vi "Trigger AI Acquisition.vi"() -> ()   [LabVIEW 2015]
doc: "이 예는 DAQmx 디바이스를 사용하여 버퍼링된 전압 측정을 연속적으로 수집하는 방법을 보여줍니다.\n\nDAQ 디바이스에 신호를 연결하는 방법에 대한 설명은 해당 디바이스 문서를 참조하십시오."
uses:
  <vilib>/DAQmx/read.llb/DAQmx Read (Analog 1D Wfm NChan NSamp).vi
  <vilib>/DAQmx/create/channels.llb/DAQmx Create Channel (AI-Voltage-Basic).vi
  <vilib>/DAQmx/configure/timing.llb/DAQmx Timing (Sample Clock).vi
  <vilib>/DAQmx/configure/task.llb/DAQmx Configure Logging (TDMS).vi
  <vilib>/DAQmx/configure/trigger.llb/DAQmx Start Trigger (Digital Edge).vi
  <vilib>/DAQmx/miscellaneous.llb/DAQmx Fill In Error Info.vi
  <resource>/objmgr/daqmx.rc
panel:
  in  "에지":i32(ring)=10280 items=["상승"=10280, "하강"=10171]
  in  "소스":tag
  in  "정지":bool
  out "웨이브폼 그래프":waveform(dbl)[](graph)
  in  "TDMS파일 경로":path
  in  "루프당 샘플":i32=1000
  in  "샘플 속도":dbl=1000.0
  in  "샘플 클럭 소스":tag="OnboardClock"
  in  "터미널 설정":i32(ring)=-1 items=["기본"=-1, "RSE"=10083, "NRSE"=10078, "차동"=10106, "유사 차동"=12529]
  in  "최대 전압":dbl=5.0
  in  "최소 전압":dbl=-5.0
  in  "물리적 채널":tag="Dev1/ai0"
  out "실제 샘플 속도":dbl=1000.0 format="%0.2f"
  in  "로깅 모드":i32(ring)=10231 items=["Off"=10231, "로그 및 읽기"=15842]
  # "채널 셋팅"
  # "수집된 데이터"
  # "트리거 셋팅"
  # "타이밍 셋팅"
  # "로깅 셋팅"
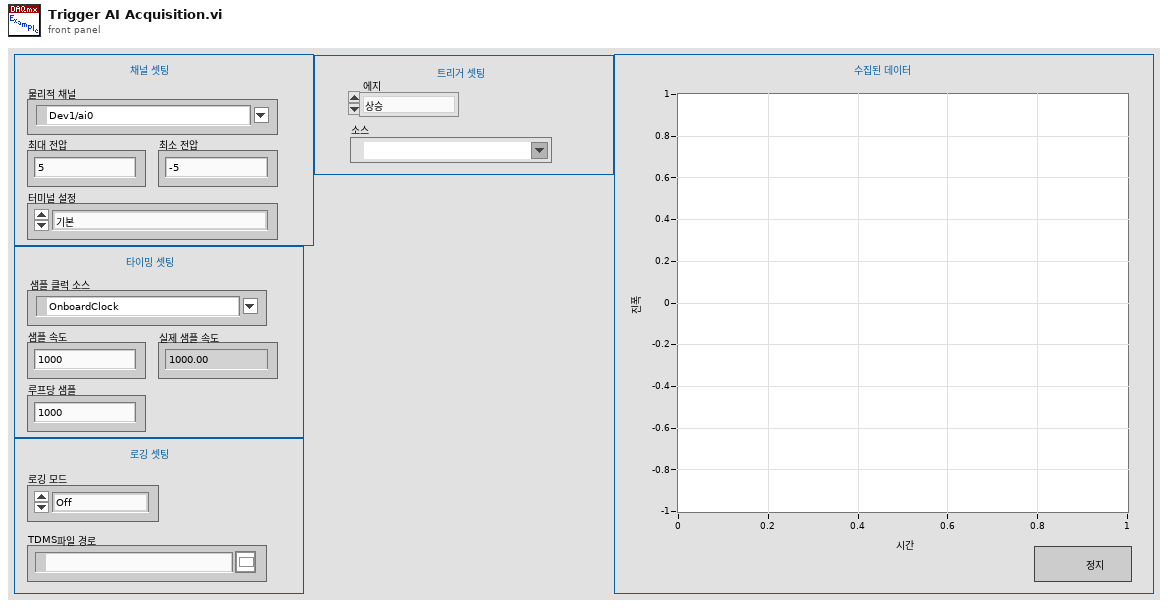
[diagram p1: front panel]
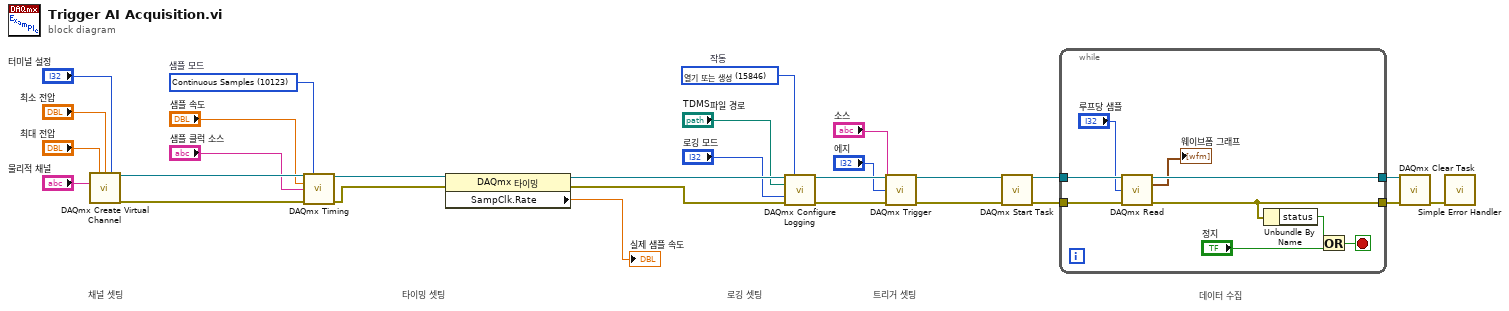
[diagram p0: block diagram]
diagram:
  w21 = 15846 items=["Open"=10437, "열기 또는 생성"=15846, "생성 또는 대체"=15847, "생성"=15848]  # 작동
  w26 = 10123 items=["유한 샘플"=10178, "Continuous Samples"=10123, "하드웨어 타이밍에 의한 단일 포인트"=12522]  # 샘플 모드
  # "트리거 셋팅"
  # "데이터 수집"
  # "타이밍 셋팅"
  # "채널 셋팅"
  # "로깅 셋팅"
  n1 = call-poly <vilib>:"DAQmx Create Virtual Channel.vi"("maximum value"="최대 전압", "minimum value"="최소 전압", "input terminal configuration"="터미널 설정", "physical channels"="물리적 채널") -> ("task out"=w24:refnum<k21>, "error out"=w25:errorcluster)  [unwired: 10 in]
  n2 = call-poly <vilib>:"DAQmx Timing.vi"("task/channels in"=w24, "sample mode"=w26, "rate"="샘플 속도", "source"="샘플 클럭 소스", "error in"=w25) -> ("task out"=w28:refnum<k21>, "error out"=w27:errorcluster)  [unwired: 9 in]
  n3 = property class="DAQmx 타이밍"(reference=w28, error in=w27) -> (reference out=w23:refnum<k21>, error out=w22:errorcluster, "SampClk.Rate"=→"실제 샘플 속도":dbl)
  n4 = call-poly <vilib>:"DAQmx Configure Logging.vi"("task/channels in"=w23, "operation"=w21, "file path"="TDMS파일 경로", "logging mode"="로깅 모드", "error in"=w22) -> ("task out"=w3:refnum<k21>, "error out"=w6:errorcluster)  [unwired: 9 in]
  n5 = call-poly <vilib>:"DAQmx Trigger.vi"("task/channels in"=w3, "source"="소스", "edge"="에지", "error in"=w6) -> ("task out"=w4:refnum<k21>, "error out"=w5:errorcluster)  [unwired: 10 in]
  n6 = call <vilib>:"DAQmx Start Task.vi"("task/channels in"=w4, "error in"=w5) -> ("task out"=w20:refnum<k21>, "error out"=w19:errorcluster)  [unwired: 12 in]
  n7 = while {
    tunnel: w20 -> [w37]
    tunnel: w19 -> [w36]
    tunnel: [w33] -> w17
    tunnel: [w34] -> w18
    stop <- w35 stop-if-true
    n8 = call-poly <vilib>:"DAQmx Read.vi"("task/channels in"=w37, "number of samples per channel"="루프당 샘플", "error in"=w36) -> ("task out"=w34:refnum<k21>, "data"=→"웨이브폼 그래프":waveform(dbl)[], "error out"=w33:errorcluster)  [unwired: 10 in]
    n9 = Unbundle By Name(w33) -> ("status"=w32:bool)
    n10 = Or(x=w32, y="정지") -> (x .or. y?=w35:bool)
  }
  n11 = call <vilib>:"DAQmx Clear Task.vi"("task in"=w18, "error in"=w17) -> ("error out"=w16:errorcluster)  [unwired: 13 in]
  n12 = call <vilib>:"Simple Error Handler.vi"("error in (no error)"=w16) -> ()  [unwired: 4 in, 5 out]
